vi "MAIN.vi"() -> ()   [LabVIEW 2017]
doc: "该模板用于创建生产者／消费者模式的应用程序，以事件驱动的方式，生成队列中的项。如需通过响应事件实现代码的异步执行，同时不影响用户界面的响应速度，可考虑用该模式替代“用户界面事件处理器”模式。"
uses:
  SubVIs/ctl/Status.ctl
  SubVIs/DataBaseModule/Sqlite/CBB/UpdateAllData.vi
  SubVIs/DataBaseModule/Sqlite/SQLite.lvlib
panel:
  out "设备Status":T1[](array[typedef])
  in  "设备明细簇":T2[](array[typedef])
  out "元素":string
  in  "选项卡控件":enum32{"主界面", "设置"}(tab)
  out "系统信息":string
  in  "关机":bool
  in  "退出":bool
  in  "自动":bool
  in  "归零":bool
  out "Status":T1
  in  "连接":bool
  in  "设备名称":T3
  in  "开机":bool
  in  "stop":bool caption="停止"
  in  "保存":bool
  in  "设备明细表格":string[][](table)
  in  "Enqueue Element":bool caption="元素入队列"
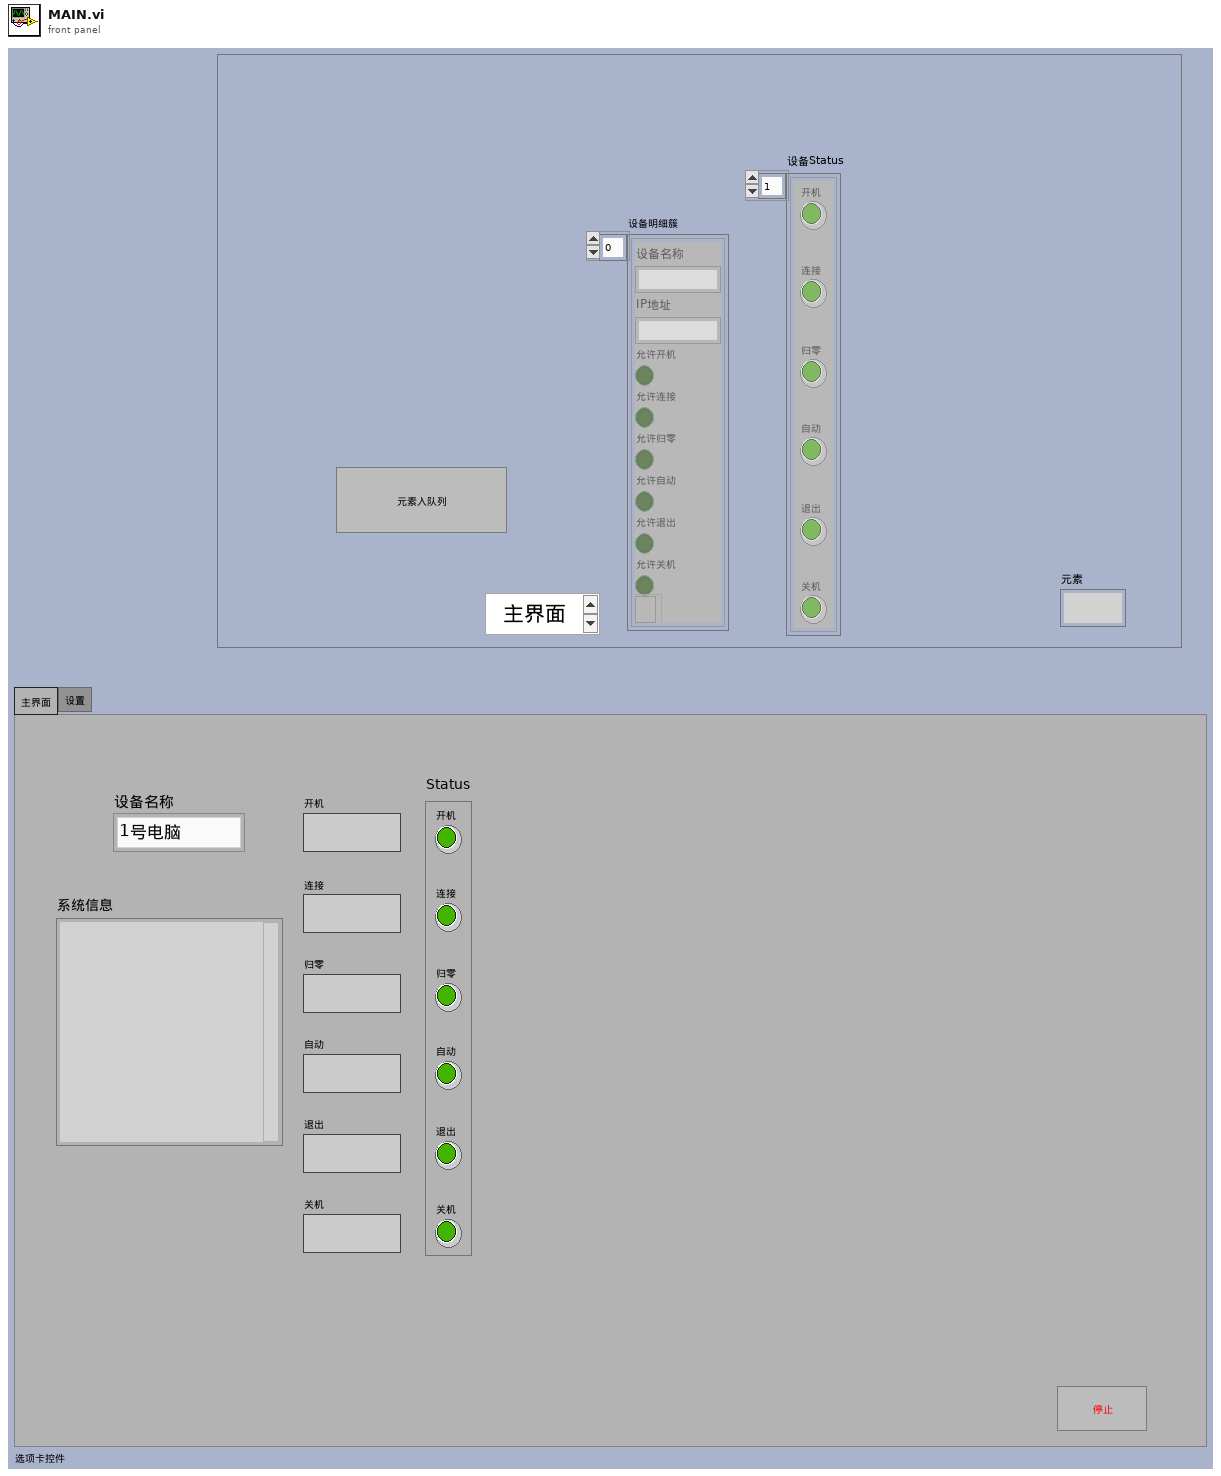
[diagram p1: front panel]
types:
  T1 = typedef "Status.ctl" = cluster{"开机":bool, "连接":bool, "归零":bool, "自动":bool, "退出":bool, "关机":bool}
  T2 = typedef "单台设备明细.ctl" = cluster{"设备名称":string, "IP地址":string, "允许开机":bool, "允许连接":bool, "允许归零":bool, "允许自动":bool, "允许退出":bool, "允许关机":bool, "connection ID":refnum<k5>}
  T3 = typedef "设备名称.ctl" = enum16{"1号电脑", "2号电脑"}
  T4 = cluster{"关机":refnum<vi>, "退出":refnum<vi>, "自动":refnum<vi>, "归零":refnum<vi>, "连接":refnum<vi>, "设备名称":refnum<vi>, "开机":refnum<vi>, "Status":refnum<vi>, "设备明细表格":refnum<vi>, "系统信息":refnum<vi>, "设备明细簇":refnum<vi>, "设备Status":refnum<vi>}
  T5 = cluster{"设备明细":cluster{"table":string, "column":string[]}, "ER":cluster{"table":string, "column":string[]}}
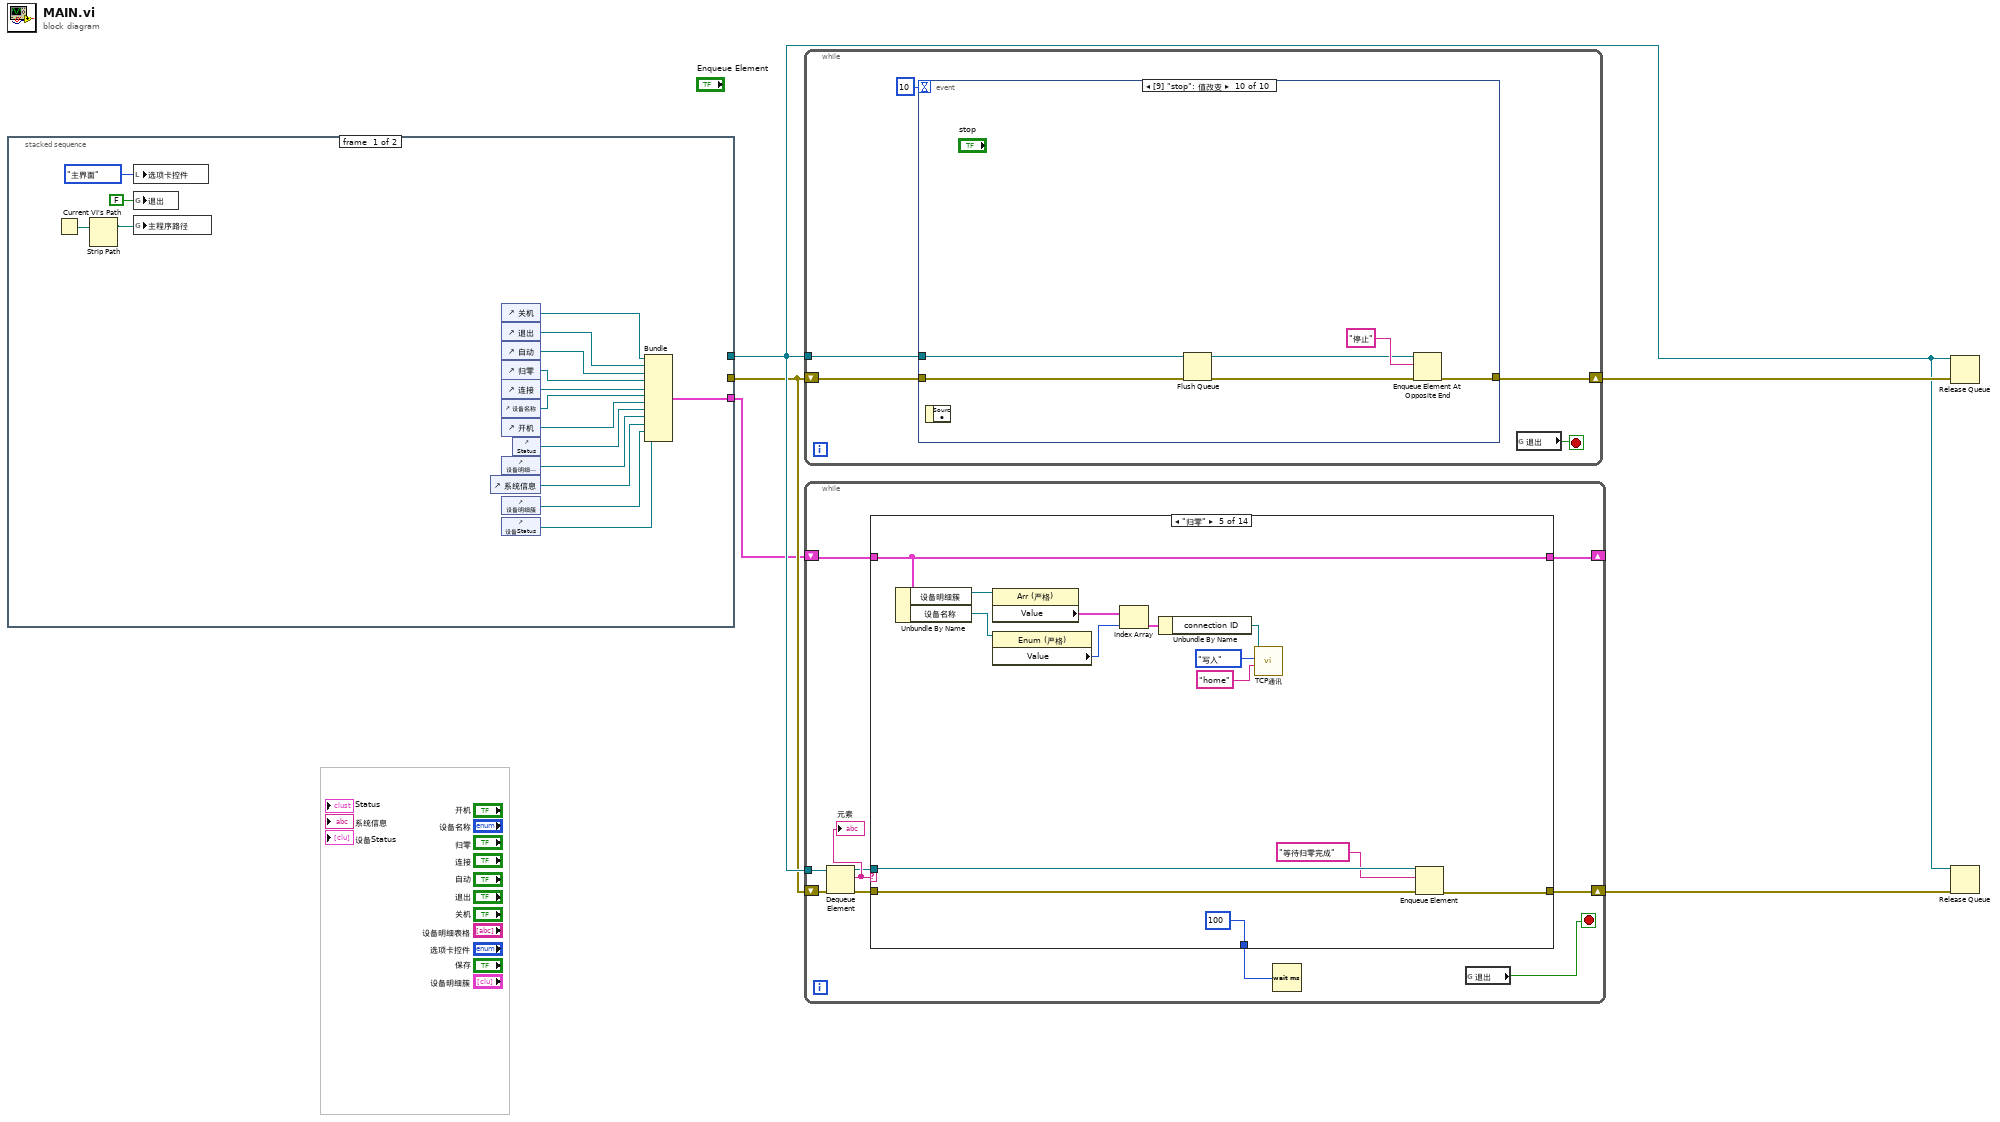
[diagram p0: block diagram]
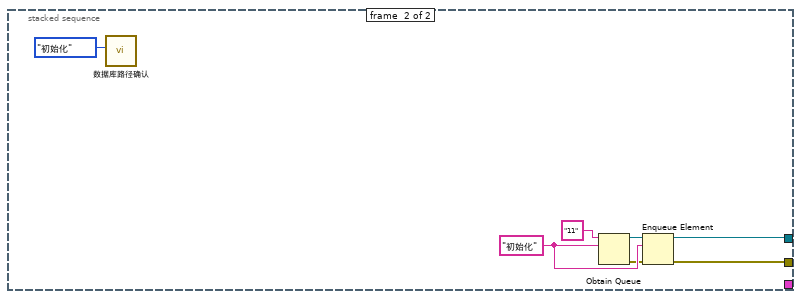
[diagram p2: hidden frame]
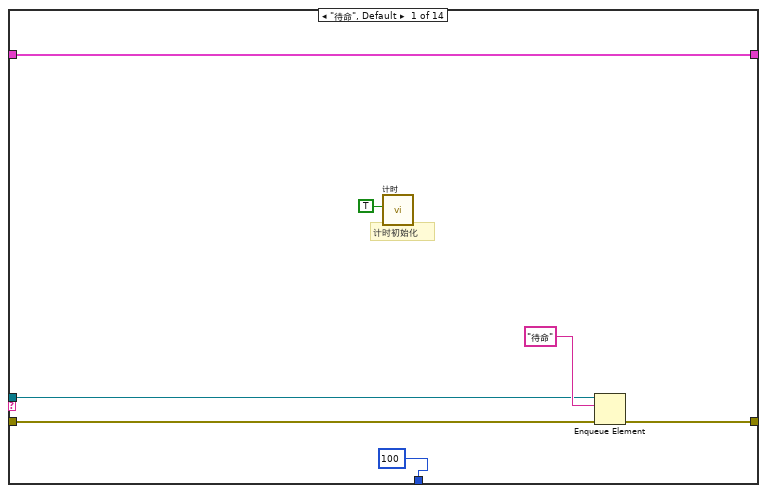
[diagram p3: hidden frame]
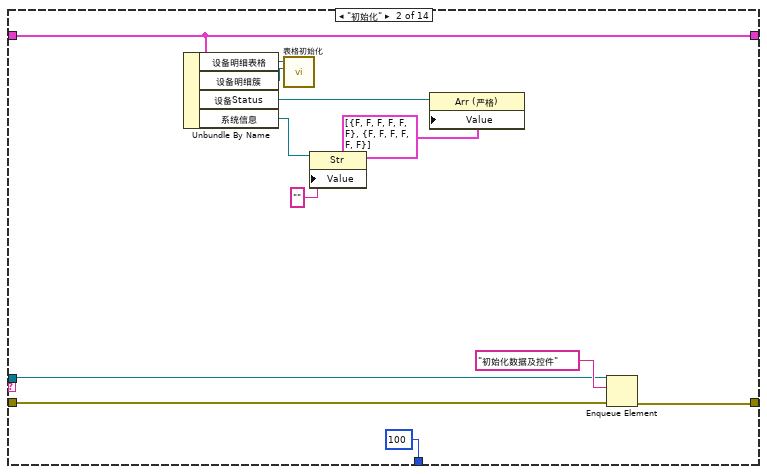
[diagram p4: hidden frame]
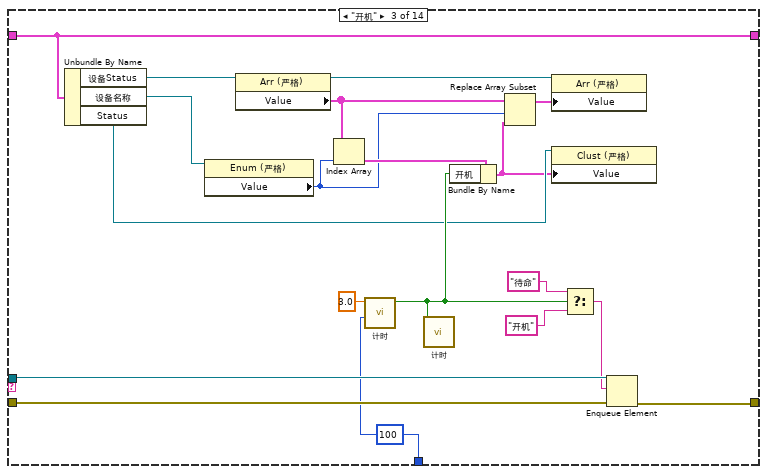
[diagram p5: hidden frame]
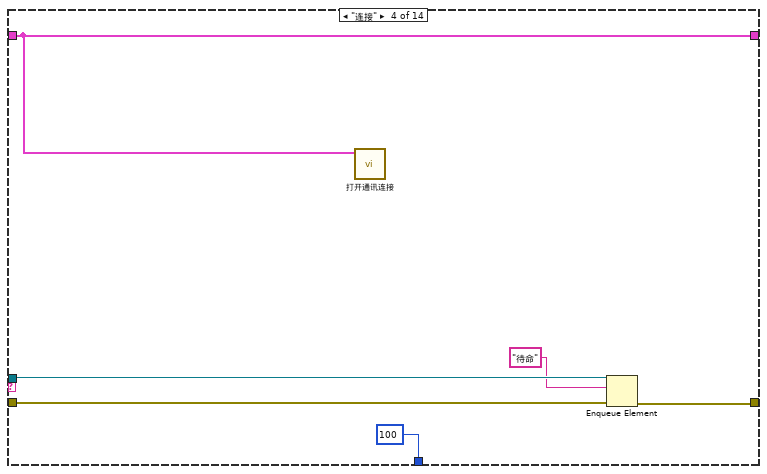
[diagram p6: hidden frame]
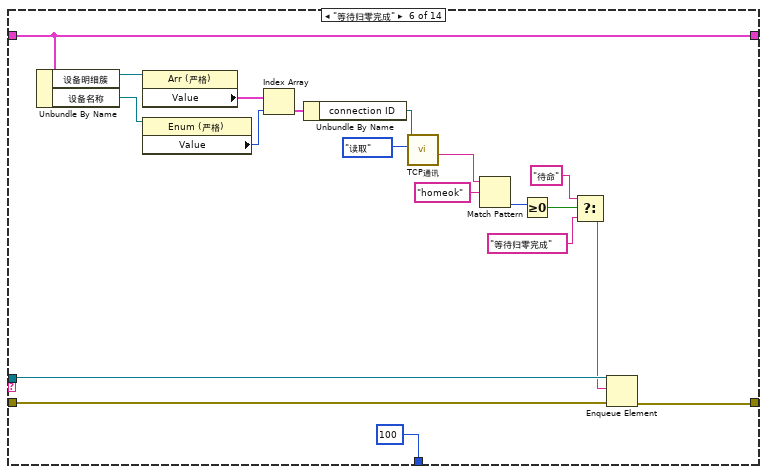
[diagram p7: hidden frame]
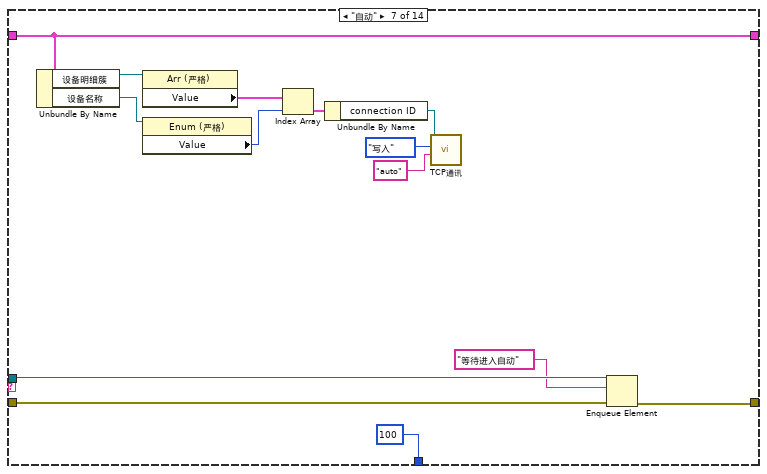
[diagram p8: hidden frame]
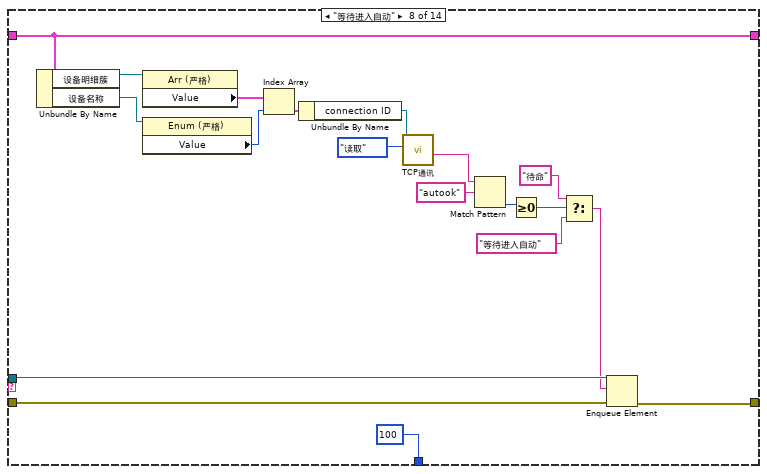
[diagram p9: hidden frame]
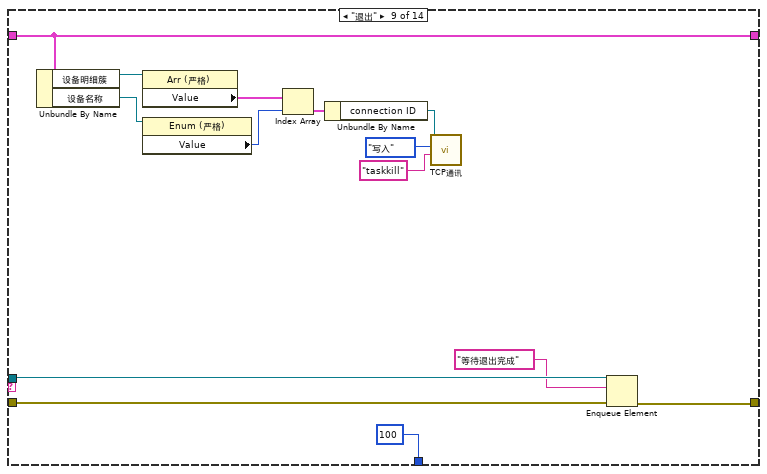
[diagram p10: hidden frame]
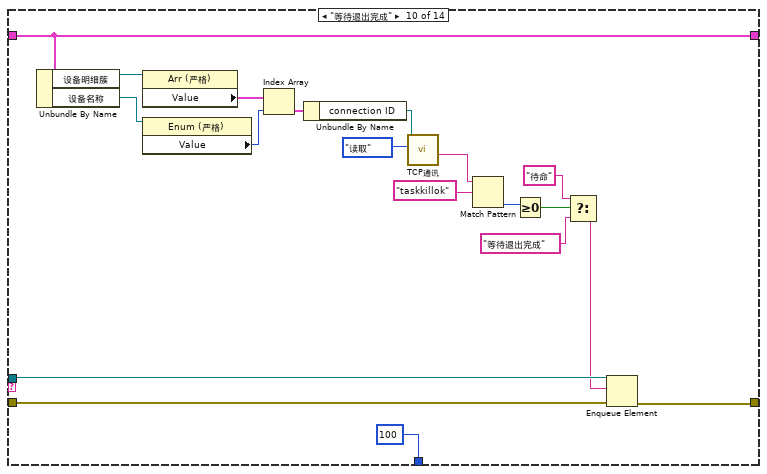
[diagram p11: hidden frame]
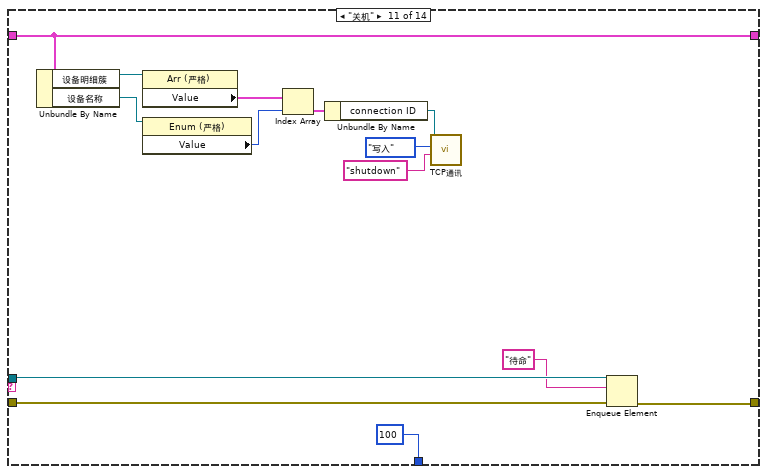
[diagram p12: hidden frame]
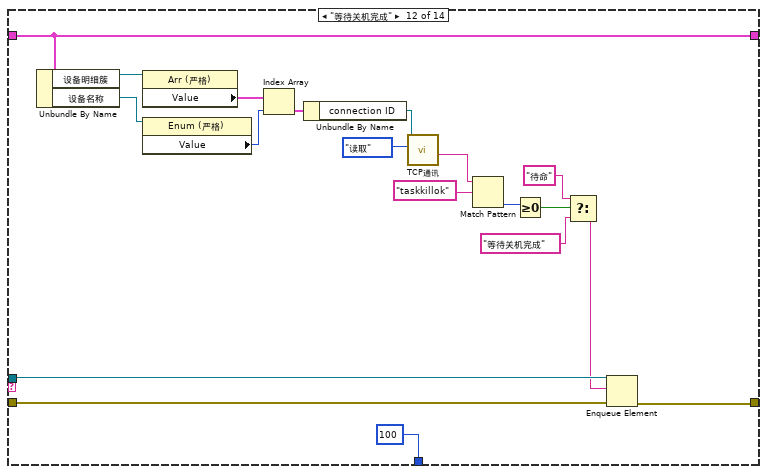
[diagram p13: hidden frame]
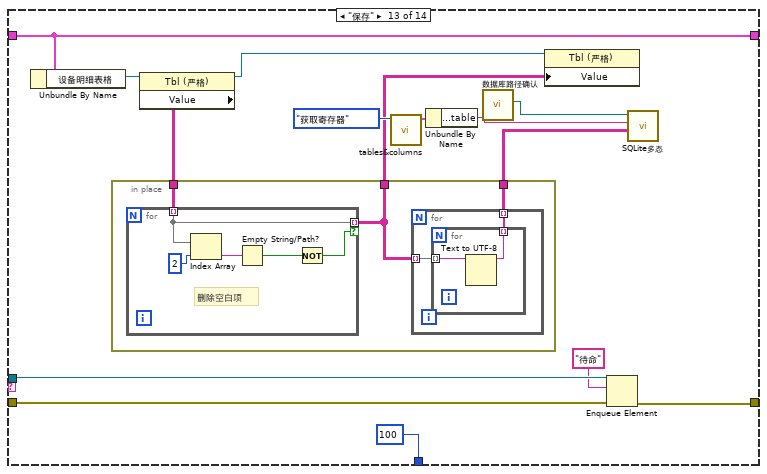
[diagram p14: hidden frame]
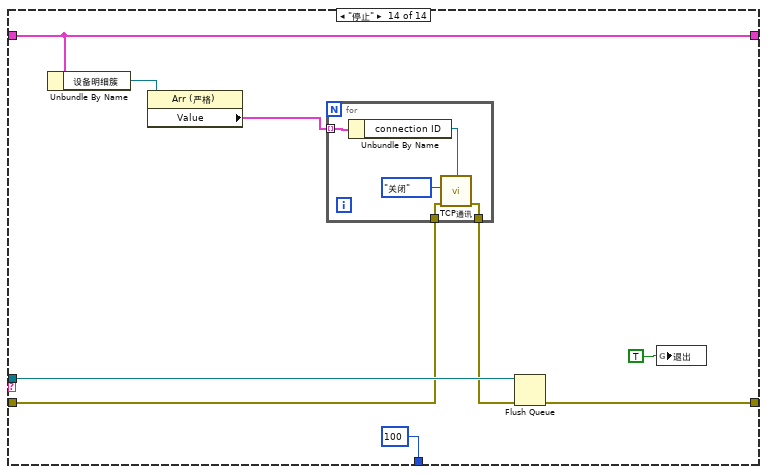
[diagram p15: hidden frame]
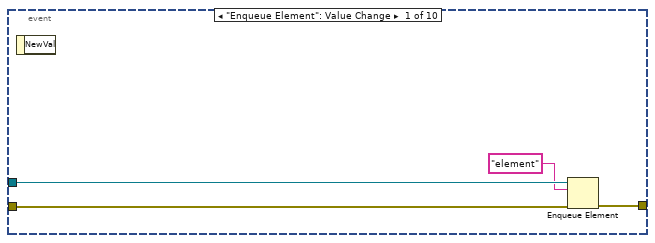
[diagram p16: hidden frame]
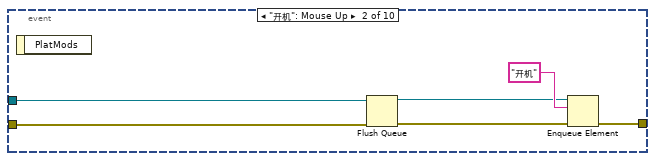
[diagram p17: hidden frame]
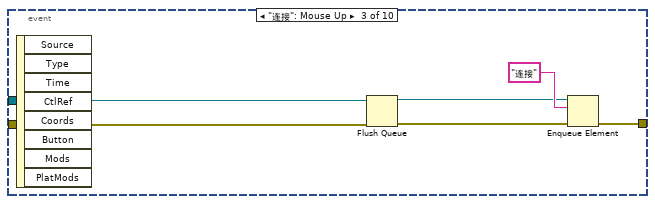
[diagram p18: hidden frame]
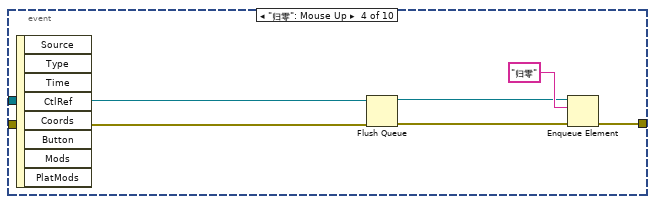
[diagram p19: hidden frame]
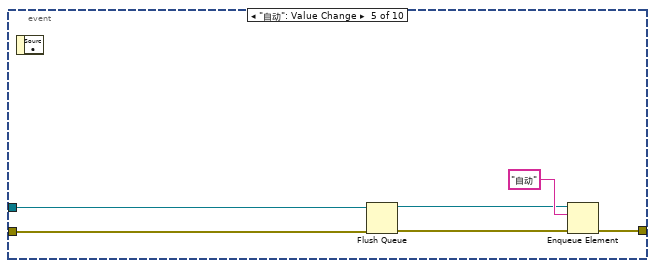
[diagram p20: hidden frame]
diagram:
  n1 = stacked-sequence {
    tunnel: [_ w24] -> w3
    tunnel: [_ w27] -> w4
    tunnel: [w12 _] -> w1
    frame #0 {
      n2 = Current VI's Path() -> (path=w10:path)
      n3 = Strip Path(path=w10) -> (stripped path=w9:path)  [unwired: 1 out]
      n4 = local write "选项卡控件"(enum32{"主界面", "设置"}."主界面" ("选项卡控件 2")) -> ()
      n5 = global write "全局 1.vi" "退出"(FALSE ("退出")) -> ()
      n6 = global write "全局 1.vi" "主程序路径"(w9) -> ()
      n7 = control-ref of="系统信息"() -> (w8:refnum<vi>)
      n8 = control-ref of="关机"() -> (w20:refnum<vi>)
      n9 = control-ref of="退出"() -> (w19:refnum<vi>)
      n10 = control-ref of="自动"() -> (w18:refnum<vi>)
      n11 = control-ref of="归零"() -> (w17:refnum<vi>)
      n12 = control-ref of="连接"() -> (w16:refnum<vi>)
      n13 = control-ref of="设备名称"() -> (w15:refnum<vi>)
      n14 = control-ref of="开机"() -> (w14:refnum<vi>)
      n15 = control-ref of="设备明细表格"() -> (w11:refnum<vi>)
      n16 = control-ref of="设备明细簇"() -> (w7:refnum<vi>)
      n17 = control-ref of="设备Status"() -> (w6:refnum<vi>)
      n18 = control-ref of="Status"() -> (w13:refnum<vi>)
      n19 = Bundle("关机"=w20, "退出"=w19, "自动"=w18, "归零"=w17, "连接"=w16, "设备名称"=w15, "开机"=w14, "Status"=w13, "设备明细表格"=w11, "系统信息"=w8, "设备明细簇"=w7, "设备Status"=w6) -> (w12:T4)  [unwired: 1 in]
    }
    frame #1 {
      w26 = "初始化"
      n20 = call "数据库路径确认.vi"("选项"=enum16{"初始化", "读取"}."初始化") -> ()  [unwired: 10 in, 1 out]
      n21 = Obtain Queue(name (unnamed)="11" ("名称（未命名）"), element data type=w26) -> (queue out=w29:refnum<queue>, error out=w25:errorcluster)  [unwired: 3 in, 1 out]
      n22 = Enqueue Element(queue=w29, element=w26, error in (no error)=w25) -> (queue out=w27:refnum<queue>, error out=w24:errorcluster)  [unwired: 1 in, 1 out]
    }
  }
  n23 = while {
    shift-right: [w32] -> w5
    shift-left: w3 -> [w33]
    tunnel: w4 -> [w34]
    stop <- w30 stop-if-true
    n24 = event shown="[9] \"stop\": 值改变" {
      selector: _ -> [_ _ _ _ _ _ _ _ _ _]
      dyn-events: _ -> [_ _ _ _ _ _ _ _ _ _]
      timeout: 10 -> [_ _ _ _ _ _ _ _ _ _]
      tunnel: w34 -> [w38 w42 w48 w54 w60 w66 w72 w78 _ w85]
      tunnel: w33 -> [w37 w40 w46 w52 w58 w64 w70 w76 _ w83]
      tunnel: [w36 w44 w50 w56 w62 w68 w74 w80 _ w82] -> w32
      event "Enqueue Element": Value Change {
        n25 = event-data() -> ()  [unwired: 1 in, 1 out]
        n26 = Enqueue Element(queue=w38, element="element", error in (no error)=w37) -> (error out=w36:errorcluster)  [unwired: 1 in, 2 out]
      }
      event "开机": Mouse Up {
        n27 = event-data() -> ()  [unwired: 1 in, 1 out]
        n28 = Flush Queue(queue=w42, error in (no error)=w40) -> (queue out=w41:refnum<queue>, error out=w39:errorcluster)  [unwired: 1 out]
        n29 = Enqueue Element(queue=w41, element="开机", error in (no error)=w39) -> (error out=w44:errorcluster)  [unwired: 1 in, 2 out]
      }
      event "连接": Mouse Up {
        n30 = event-data() -> ()  [unwired: 1 in, 8 out]
        n31 = Flush Queue(queue=w48, error in (no error)=w46) -> (queue out=w47:refnum<queue>, error out=w45:errorcluster)  [unwired: 1 out]
        n32 = Enqueue Element(queue=w47, element="连接", error in (no error)=w45) -> (error out=w50:errorcluster)  [unwired: 1 in, 2 out]
      }
      event "归零": Mouse Up {
        n33 = event-data() -> ()  [unwired: 1 in, 8 out]
        n34 = Flush Queue(queue=w54, error in (no error)=w52) -> (queue out=w53:refnum<queue>, error out=w51:errorcluster)  [unwired: 1 out]
        n35 = Enqueue Element(queue=w53, element="归零", error in (no error)=w51) -> (error out=w56:errorcluster)  [unwired: 1 in, 2 out]
      }
      event "自动": Value Change {
        n36 = event-data() -> ()  [unwired: 1 in, 1 out]
        n37 = Flush Queue(queue=w60, error in (no error)=w58) -> (queue out=w59:refnum<queue>, error out=w57:errorcluster)  [unwired: 1 out]
        n38 = Enqueue Element(queue=w59, element="自动", error in (no error)=w57) -> (error out=w62:errorcluster)  [unwired: 1 in, 2 out]
      }
      event "退出": Mouse Up {
        n39 = event-data() -> ()  [unwired: 1 in, 1 out]
        n40 = Flush Queue(queue=w66, error in (no error)=w64) -> (queue out=w65:refnum<queue>, error out=w63:errorcluster)  [unwired: 1 out]
        n41 = Enqueue Element(queue=w65, element="退出", error in (no error)=w63) -> (error out=w68:errorcluster)  [unwired: 1 in, 2 out]
      }
      event "关机": Mouse Up {
        n42 = event-data() -> ()  [unwired: 1 in, 1 out]
        n43 = Flush Queue(queue=w72, error in (no error)=w70) -> (queue out=w71:refnum<queue>, error out=w69:errorcluster)  [unwired: 1 out]
        n44 = Enqueue Element(queue=w71, element="关机", error in (no error)=w69) -> (error out=w74:errorcluster)  [unwired: 1 in, 2 out]
      }
      event "保存": Mouse Up {
        n45 = event-data() -> ()  [unwired: 1 in, 1 out]
        n46 = Flush Queue(queue=w78, error in (no error)=w76) -> (queue out=w77:refnum<queue>, error out=w75:errorcluster)  [unwired: 1 out]
        n47 = Enqueue Element(queue=w77, element="保存", error in (no error)=w75) -> (error out=w80:errorcluster)  [unwired: 1 in, 2 out]
      }
      event Timeout {
        n48 = event-data() -> ()  [unwired: 1 in, 3 out]
      }
      event "stop": Value Change {
        n49 = event-data() -> ()  [unwired: 1 in, 1 out]
        n50 = Flush Queue(queue=w85) -> (queue out=w81:refnum<queue>)  [unwired: 1 in, 2 out]
        n51 = Enqueue Element At Opposite End(queue=w81, element="停止" ("元素"), error in (no error)=w83) -> (error out=w82:errorcluster)  [unwired: 1 in, 2 out]
      }
    }
    n52 = global read "全局 1.vi" "退出"() -> (w30:bool)
  }
  n53 = while {
    shift-right: [w91] -> _
    shift-left: w1 -> [w90]
    tunnel: w4 -> [w95]
    shift-right: [w88] -> w2
    shift-left: w3 -> [w89]
    stop <- w87 stop-if-true
    n54 = Dequeue Element(queue=w95, error in (no error)=w89) -> (queue out=w92:refnum<queue>, element=w94:string, error out=w93:errorcluster)  [unwired: 1 in, 1 out]
    "元素" <- w94
    n55 = case shown="\"归零\"" w94 {
      tunnel: w93 -> [w99 w114 w133 w139 w153 w172 w186 w205 w219 w238 w252 w271 w286 w300]
      tunnel: [w97 w112 w132 w138 w152 w171 w185 w204 w218 w237 w251 w270 w285 w306] -> w88
      tunnel: w92 -> [w98 w111 w131 w137 w151 w170 w184 w203 w217 w236 w250 w269 w284 w307]
      tunnel: [w102 w109 w125 w134 w148 w168 w181 w201 w214 w234 w247 w267 w279 w303] -> w91
      tunnel: w90 -> [w102 w109 w125 w134 w148 w168 w181 w201 w214 w234 w247 w267 w279 w303]
      tunnel: [u32 100 ("等待时间（毫秒）") u32 100 ("等待时间（毫秒）") w128 u32 100 ("等待时间（毫秒）") u32 100 ("等待时间（毫秒）") u32 100 ("等待时间（毫秒）") u32 100 ("等待时间（毫秒）") u32 100 ("等待时间（毫秒）") u32 100 ("等待时间（毫秒）") u32 100 ("等待时间（毫秒）") u32 100 ("等待时间（毫秒）") u32 100 ("等待时间（毫秒）") u32 100 ("等待时间（毫秒）") u32 100 ("等待时间（毫秒）")] -> w86
      frame "待命", Default {
        # "计时初始化"
        n56 = call "计时.vi"("初始化"=TRUE) -> ()  [unwired: 9 in, 2 out]
        n57 = Enqueue Element(queue=w98, element="待命", error in (no error)=w99) -> (error out=w97:errorcluster)  [unwired: 1 in, 2 out]
      }
      frame "初始化" {
        n58 = Unbundle By Name(w109) -> ("设备明细表格"=w108:refnum<vi>, "设备明细簇"=w107:refnum<vi>, "设备Status"=w106:refnum<vi>, "系统信息"=w104:refnum<vi>)
        n59 = call "表格初始化.vi"("设备明细簇"=w107, "Table输入"=w108) -> ()  [unwired: 10 in]
        n60 = property class="Str"(reference=w104, "Value"="" ("值")) -> ()  [unwired: 1 in, 2 out]
        n61 = property class="Arr (严格)"(reference=w106, "Value"=T1[] [{"开机"=FALSE, "连接"=FALSE, "归零"=FALSE, "自动"=FALSE, "退出"=FALSE, "关机"=FALSE}, {"开机"=FALSE, "连接"=FALSE, "归零"=FALSE, "自动"=FALSE, "退出"=FALSE, "关机"=FALSE}] ("值")) -> ()  [unwired: 1 in, 2 out]
        n62 = Enqueue Element(queue=w111, element="初始化数据及控件", error in (no error)=w114) -> (error out=w112:errorcluster)  [unwired: 1 in, 2 out]
      }
      frame "开机" {
        w128 = u32 100 ("等待时间（毫秒）")
        n63 = Unbundle By Name(w125) -> ("设备Status"=w124:refnum<vi>, "设备名称"=w123:refnum<vi>, "Status"=w116:refnum<vi>)
        n64 = property class="Enum (严格)"(reference=w123) -> ("Value"=w119:T3)  [unwired: 1 in, 2 out]
        n65 = property class="Arr (严格)"(reference=w124) -> (reference out=w118:refnum<vi>, "Value"=w120:T1[])  [unwired: 1 in, 1 out]
        n66 = Index Array(array=w120, index=w119) -> (element=w122:T1)
        n67 = call "计时.vi"("单位"=w128, "计时时间(s)"=3.0) -> ("完成"=w121:bool)  [unwired: 8 in, 1 out]
        n68 = call "计时.vi"("初始化"=w121) -> ()  [unwired: 9 in, 2 out]
        n69 = Bundle By Name(cluster=w122, "开机"=w121) -> (w115:T1)
        n70 = Replace Array Subset(array=w120, new element=w115, index=w119) -> (w117:T1[])
        n71 = property class="Arr (严格)"(reference=w118, "Value"=w117) -> ()  [unwired: 1 in, 2 out]
        n72 = property class="Clust (严格)"(reference=w116, "Value"=w115) -> ()  [unwired: 1 in, 2 out]
        n73 = Select(t="待命", s=w121, f="开机" ("element")) -> (s? t:f=w126:string)
        n74 = Enqueue Element(queue=w131, element=w126, error in (no error)=w133) -> (error out=w132:errorcluster)  [unwired: 1 in, 2 out]
      }
      frame "连接" {
        n75 = call "打开通讯连接.vi"("簇"=w134) -> ()  [unwired: 11 in]
        n76 = Enqueue Element(queue=w137, element="待命" ("t"), error in (no error)=w139) -> (error out=w138:errorcluster)  [unwired: 1 in, 2 out]
      }
      frame "归零" {
        n77 = Unbundle By Name(w148) -> ("设备明细簇"=w147:refnum<vi>, "设备名称"=w145:refnum<vi>)
        n78 = property class="Arr (严格)"(reference=w147) -> ("Value"=w143:T2[])  [unwired: 1 in, 2 out]
        n79 = property class="Enum (严格)"(reference=w145) -> ("Value"=w142:T3)  [unwired: 1 in, 2 out]
        n80 = Index Array(array=w143, index=w142) -> (element=w144:T2)
        n81 = Unbundle By Name(w144) -> ("connection ID"=w141:refnum<k5>)
        n82 = call "TCP通讯.vi"("数据输入"="home", "选项"=enum16{"NA", "侦听", "读取", "写入", "关闭"}."写入", "connection ID in"=w141) -> ()  [unwired: 4 in, 5 out]
        n83 = Enqueue Element(queue=w151, element="等待归零完成" ("t"), error in (no error)=w153) -> (error out=w152:errorcluster)  [unwired: 1 in, 2 out]
      }
      frame "等待归零完成" {
        n84 = Unbundle By Name(w168) -> ("设备明细簇"=w167:refnum<vi>, "设备名称"=w165:refnum<vi>)
        n85 = property class="Arr (严格)"(reference=w167) -> ("Value"=w163:T2[])  [unwired: 1 in, 2 out]
        n86 = property class="Enum (严格)"(reference=w165) -> ("Value"=w162:T3)  [unwired: 1 in, 2 out]
        n87 = Index Array(array=w163, index=w162) -> (element=w164:T2)
        n88 = Unbundle By Name(w164) -> ("connection ID"=w161:refnum<k5>)
        n89 = call "TCP通讯.vi"("选项"=enum16{"NA", "侦听", "读取", "写入", "关闭"}."读取", "connection ID in"=w161) -> ("数据输出"=w160:string)  [unwired: 5 in, 4 out]
        n90 = Match Pattern(string=w160, regular expression="homeok" ("正则表达式")) -> (offset past match=w158:i32)  [unwired: 1 in, 3 out]
        n91 = Greater Or Equal To 0?(x=w158) -> (x >= 0?=w157:bool)
        n92 = Select(t="待命", s=w157, f="等待归零完成" ("t")) -> (s? t:f=w155:string)
        n93 = Enqueue Element(queue=w170, element=w155, error in (no error)=w172) -> (error out=w171:errorcluster)  [unwired: 1 in, 2 out]
      }
      frame "自动" {
        n94 = Unbundle By Name(w181) -> ("设备明细簇"=w180:refnum<vi>, "设备名称"=w178:refnum<vi>)
        n95 = property class="Arr (严格)"(reference=w180) -> ("Value"=w176:T2[])  [unwired: 1 in, 2 out]
        n96 = property class="Enum (严格)"(reference=w178) -> ("Value"=w175:T3)  [unwired: 1 in, 2 out]
        n97 = Index Array(array=w176, index=w175) -> (element=w177:T2)
        n98 = Unbundle By Name(w177) -> ("connection ID"=w174:refnum<k5>)
        n99 = call "TCP通讯.vi"("数据输入"="auto", "选项"=enum16{"NA", "侦听", "读取", "写入", "关闭"}."写入", "connection ID in"=w174) -> ()  [unwired: 4 in, 5 out]
        n100 = Enqueue Element(queue=w184, element="等待进入自动" ("t"), error in (no error)=w186) -> (error out=w185:errorcluster)  [unwired: 1 in, 2 out]
      }
      frame "等待进入自动" {
        n101 = Unbundle By Name(w201) -> ("设备明细簇"=w200:refnum<vi>, "设备名称"=w198:refnum<vi>)
        n102 = property class="Arr (严格)"(reference=w200) -> ("Value"=w196:T2[])  [unwired: 1 in, 2 out]
        n103 = property class="Enum (严格)"(reference=w198) -> ("Value"=w195:T3)  [unwired: 1 in, 2 out]
        n104 = Index Array(array=w196, index=w195) -> (element=w197:T2)
        n105 = Unbundle By Name(w197) -> ("connection ID"=w194:refnum<k5>)
        n106 = call "TCP通讯.vi"("选项"=enum16{"NA", "侦听", "读取", "写入", "关闭"}."读取", "connection ID in"=w194) -> ("数据输出"=w193:string)  [unwired: 5 in, 4 out]
        n107 = Match Pattern(string=w193, regular expression="autook" ("正则表达式")) -> (offset past match=w191:i32)  [unwired: 1 in, 3 out]
        n108 = Greater Or Equal To 0?(x=w191) -> (x >= 0?=w190:bool)
        n109 = Select(t="待命", s=w190, f="等待进入自动" ("t")) -> (s? t:f=w188:string)
        n110 = Enqueue Element(queue=w203, element=w188, error in (no error)=w205) -> (error out=w204:errorcluster)  [unwired: 1 in, 2 out]
      }
      frame "退出" {
        n111 = Unbundle By Name(w214) -> ("设备明细簇"=w213:refnum<vi>, "设备名称"=w211:refnum<vi>)
        n112 = property class="Arr (严格)"(reference=w213) -> ("Value"=w209:T2[])  [unwired: 1 in, 2 out]
        n113 = property class="Enum (严格)"(reference=w211) -> ("Value"=w208:T3)  [unwired: 1 in, 2 out]
        n114 = Index Array(array=w209, index=w208) -> (element=w210:T2)
        n115 = Unbundle By Name(w210) -> ("connection ID"=w207:refnum<k5>)
        n116 = call "TCP通讯.vi"("数据输入"="taskkill", "选项"=enum16{"NA", "侦听", "读取", "写入", "关闭"}."写入", "connection ID in"=w207) -> ()  [unwired: 4 in, 5 out]
        n117 = Enqueue Element(queue=w217, element="等待退出完成" ("t"), error in (no error)=w219) -> (error out=w218:errorcluster)  [unwired: 1 in, 2 out]
      }
      frame "等待退出完成" {
        n118 = Unbundle By Name(w234) -> ("设备明细簇"=w233:refnum<vi>, "设备名称"=w231:refnum<vi>)
        n119 = property class="Arr (严格)"(reference=w233) -> ("Value"=w229:T2[])  [unwired: 1 in, 2 out]
        n120 = property class="Enum (严格)"(reference=w231) -> ("Value"=w228:T3)  [unwired: 1 in, 2 out]
        n121 = Index Array(array=w229, index=w228) -> (element=w230:T2)
        n122 = Unbundle By Name(w230) -> ("connection ID"=w227:refnum<k5>)
        n123 = call "TCP通讯.vi"("选项"=enum16{"NA", "侦听", "读取", "写入", "关闭"}."读取", "connection ID in"=w227) -> ("数据输出"=w226:string)  [unwired: 5 in, 4 out]
        n124 = Match Pattern(string=w226, regular expression="taskkillok" ("正则表达式")) -> (offset past match=w224:i32)  [unwired: 1 in, 3 out]
        n125 = Greater Or Equal To 0?(x=w224) -> (x >= 0?=w223:bool)
        n126 = Select(t="待命", s=w223, f="等待退出完成" ("t")) -> (s? t:f=w221:string)
        n127 = Enqueue Element(queue=w236, element=w221, error in (no error)=w238) -> (error out=w237:errorcluster)  [unwired: 1 in, 2 out]
      }
      frame "关机" {
        n128 = Unbundle By Name(w247) -> ("设备明细簇"=w246:refnum<vi>, "设备名称"=w244:refnum<vi>)
        n129 = property class="Arr (严格)"(reference=w246) -> ("Value"=w242:T2[])  [unwired: 1 in, 2 out]
        n130 = property class="Enum (严格)"(reference=w244) -> ("Value"=w241:T3)  [unwired: 1 in, 2 out]
        n131 = Index Array(array=w242, index=w241) -> (element=w243:T2)
        n132 = Unbundle By Name(w243) -> ("connection ID"=w240:refnum<k5>)
        n133 = call "TCP通讯.vi"("数据输入"="shutdown", "选项"=enum16{"NA", "侦听", "读取", "写入", "关闭"}."写入", "connection ID in"=w240) -> ()  [unwired: 4 in, 5 out]
        n134 = Enqueue Element(queue=w250, element="待命" ("t"), error in (no error)=w252) -> (error out=w251:errorcluster)  [unwired: 1 in, 2 out]
      }
      frame "等待关机完成" {
        n135 = Unbundle By Name(w267) -> ("设备明细簇"=w266:refnum<vi>, "设备名称"=w264:refnum<vi>)
        n136 = property class="Arr (严格)"(reference=w266) -> ("Value"=w262:T2[])  [unwired: 1 in, 2 out]
        n137 = property class="Enum (严格)"(reference=w264) -> ("Value"=w261:T3)  [unwired: 1 in, 2 out]
        n138 = Index Array(array=w262, index=w261) -> (element=w263:T2)
        n139 = Unbundle By Name(w263) -> ("connection ID"=w260:refnum<k5>)
        n140 = call "TCP通讯.vi"("选项"=enum16{"NA", "侦听", "读取", "写入", "关闭"}."读取", "connection ID in"=w260) -> ("数据输出"=w259:string)  [unwired: 5 in, 4 out]
        n141 = Match Pattern(string=w259, regular expression="taskkillok" ("正则表达式")) -> (offset past match=w257:i32)  [unwired: 1 in, 3 out]
        n142 = Greater Or Equal To 0?(x=w257) -> (x >= 0?=w256:bool)
        n143 = Select(t="待命", s=w256, f="等待关机完成" ("t")) -> (s? t:f=w254:string)
        n144 = Enqueue Element(queue=w269, element=w254, error in (no error)=w271) -> (error out=w270:errorcluster)  [unwired: 1 in, 2 out]
      }
      frame "保存" {
        n145 = Unbundle By Name(w279) -> ("设备明细表格"=w281:refnum<vi>)
        n146 = property class="Tbl (严格)"(reference=w281) -> (reference out=w278:refnum<vi>, "Value"=w277:string[][])  [unwired: 1 in, 1 out]
        n147 = in-place {
          in-place-border: w277 -> [w289]
          in-place-border: [w288] -> w273
          in-place-border: [w287] -> w272
          n148 = for {
            tunnel: w289 -> [w298] mode=indexing
            tunnel: [w298] -> w288 mode=indexing if=w294
            # "删除空白项"
            n149 = Index Array(array=w298, index=2 ("禁用的索引 (列)")) -> (element=w296:string)
            n150 = Empty String/Path?(string/path=w296) -> (empty?=w295:bool)
            n151 = Not(x=w295) -> (.not. x?=w294:bool)
          }
          n152 = for {
            tunnel: w288 -> [w291] mode=indexing
            tunnel: [w290] -> w287 mode=indexing
            n153 = for {
              tunnel: w291 -> [w293] mode=indexing
              tunnel: [w292] -> w290 mode=indexing
              n154 = Text to UTF-8(11:w293) -> (3:w292:string)  [unwired: 2 in, 1 out]
            }
          }
        }
        n155 = call "tables&columns.vi"("选项"=enum16{"初始化", "获取寄存器"}."获取寄存器") -> ("Tables&columns"=w275:T5)  [unwired: 9 in, 1 out]
        n156 = Unbundle By Name(w275) -> ("设备明细.table"=w274:string)
        n157 = call "数据库路径确认.vi"() -> ("数据库路径"=w280:path)  [unwired: 11 in]
        n158 = property class="Tbl (严格)"(reference=w278, "Value"=w273) -> ()  [unwired: 1 in, 2 out]
        n159 = Enqueue Element(queue=w284, element="待命" ("t"), error in (no error)=w286) -> (error out=w285:errorcluster)  [unwired: 1 in, 2 out]
        n160 = call-poly "SQLite多态.vi"("AllData"=w272, "Table Name"=w274, "DbPath"=w280) -> ()  [unwired: 5 in, 4 out]
      }
      frame "停止" {
        n161 = Unbundle By Name(w303) -> ("设备明细簇"=w302:refnum<vi>)
        n162 = property class="Arr (严格)"(reference=w302) -> ("Value"=w301:T2[])  [unwired: 1 in, 2 out]
        n163 = for {
          tunnel: w301 -> [w311] mode=indexing
          tunnel: w300 -> [w309]
          tunnel: [w308] -> w299
          n164 = Unbundle By Name(w311) -> ("connection ID"=w310:refnum<k5>)
          n165 = call "TCP通讯.vi"("error in"=w309, "选项"=enum16{"NA", "侦听", "读取", "写入", "关闭"}."关闭", "connection ID in"=w310) -> ("error out"=w308:errorcluster)  [unwired: 4 in, 4 out]
        }
        n166 = Flush Queue(queue=w307, error in (no error)=w299) -> (error out=w306:errorcluster)  [unwired: 2 out]
        n167 = global write "全局 1.vi" "退出"(TRUE) -> ()
      }
    }
    n168 = Wait (ms)(milliseconds to wait=w86) -> ()  [unwired: 1 out]
    n169 = global read "全局 1.vi" "退出"() -> (w87:bool)
  }
  n170 = Release Queue(queue=w4, error in (no error)=w5) -> ()  [unwired: 1 in, 3 out]
  n171 = Release Queue(queue=w4, error in (no error)=w2) -> ()  [unwired: 1 in, 3 out]
